vi "Copy .LVLIBP to NI VeriStand dir.vi"(8 "error in (no error)":errorcluster, 9 "CD name":string="FPGA Addon", 10 "CD Folder name":string="Custom Devices", 11 "Project Path":path) -> (0 "error out":errorcluster)   [LabVIEW 2021, in "LVLIBP CD XML Updater.lvlib"]
doc: "This VI is called after each run of a build specification. The VI will copy the generated LLB (Engine or System Explorer) into the VeriStand Custom Device folder (...\\Documents\\National Instruments\\NI VeriStand 2013...)."
uses:
  LVLIBP CD XML Updater.lvlib
  <vilib>/Utility/sysdir.llb/System Directory Type.ctl
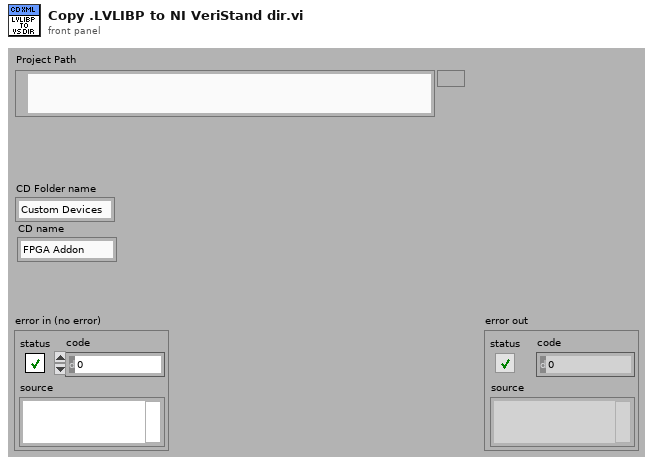
[diagram p1: front panel]
types:
  T1 = typedef "System Directory Type.ctl" = i32
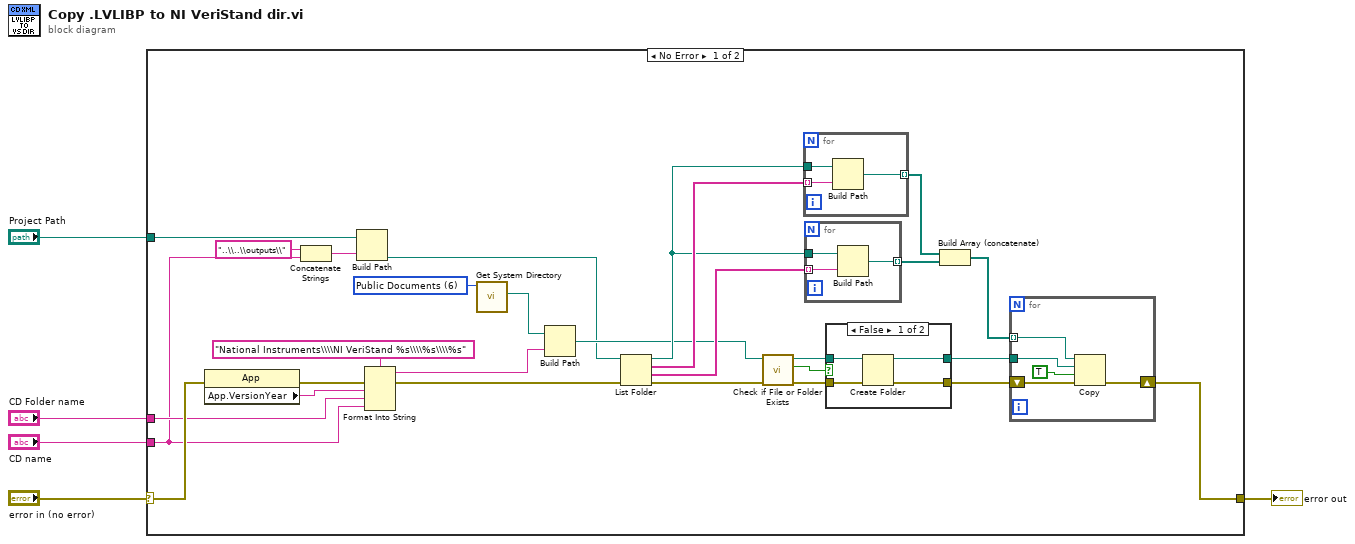
[diagram p0: block diagram]
diagram:
  n1 = case shown="No Error" "error in (no error)" {
    selector: "error in (no error)" -> [w16 w51]
    tunnel: [w18 w51] -> w3
    tunnel: "Project Path" -> [w14 _]
    tunnel: "CD Folder name" -> [w10 _]
    tunnel: "CD name" -> [w7 _]
    frame No Error {
      w21 = T1 6 items=["User Home"=0, "User Desktop"=1, "User Documents"=2, "User Application Data"=3, "User Preferences"=4, "User Temporary"=5, "Public Documents"=6, "Public Application Data"=7, "Public Preferences"=8, "Public Cache"=13, "System Core Libraries"=9, "System Installed Libraries"=10, "Application Files"=11, "Boot Volume Root"=12] ("system directory type")
      n2 = property class="App"(error in=w16) -> (error out=w20:errorcluster, "App.VersionYear"=w19:string)  [unwired: 1 in, 1 out]
      n3 = Concatenate Strings("..\\..\\outputs\\" ("string"), w7) -> (w6:string)
      n4 = Build Path(base path=w14, name or relative path=w6) -> (appended path=w11:path)
      n5 = Format Into String(format string="National Instruments\\\\NI VeriStand %s\\\\%s\\\\%s" ("name or relative path"), error in=w20, w19, w10, w7) -> (resulting string=w23:string, error out=w15:errorcluster)  [unwired: 1 in]
      n6 = call <vilib>:"Get System Directory.vi"("system directory type"=w21) -> ("system directory"=w22:path)  [unwired: 10 in]
      n7 = Build Path(base path=w22, name or relative path=w23) -> (appended path=w17:path)
      n8 = List Folder(path=w11, error in=w15) -> (path out=w26:path, filenames=w33:string[], folder names=w27:string[], error out=w24:errorcluster)  [unwired: 2 in]
      n9 = call <vilib>:"Check if File or Folder Exists.vi"("error in (no error)"=w24, "path"=w17) -> ("error out"=w28:errorcluster, "file or folder exists?"=w30:bool, "dup path"=w29:path)  [unwired: 7 in]
      n10 = for {
        tunnel: w33 -> [w49] mode=indexing
        tunnel: w26 -> [w50]
        tunnel: [w48] -> w32 mode=indexing
        n11 = Build Path(base path=w50, name or relative path=w49) -> (appended path=w48:path)
      }
      n12 = for {
        tunnel: w27 -> [w46] mode=indexing
        tunnel: w26 -> [w47]
        tunnel: [w45] -> w25 mode=indexing
        n13 = Build Path(base path=w47, name or relative path=w46) -> (appended path=w45:path)
      }
      n14 = case shown="False" w30 {
        tunnel: w29 -> [w37 w39]
        tunnel: w28 -> [w36 w38]
        tunnel: [w35 w39] -> w13
        tunnel: [w34 w38] -> w12
        frame False {
          n15 = Create Folder(path (use dialog)=w37, error in=w36) -> (created path=w35:path, error out=w34:errorcluster)  [unwired: 1 in, 1 out]
        }
        frame True {
        }
      }
      n16 = Build Array (concatenate)(w32, w25) -> (w31:path[])
      n17 = for {
        tunnel: w31 -> [w41] mode=indexing
        shift-right: [w42] -> w18
        shift-left: w12 -> [w43]
        tunnel: w13 -> [w40]
        n18 = Copy(8:w43, 9:TRUE ("overwrite (F)"), 10:w40, 11:w41) -> (0:w42:errorcluster)  [unwired: 1 in, 2 out]
      }
    }
    frame Error {
    }
  }
  "error out" <- w3
